vi "HGF_PVBase.appendData2Variant.vi"(0 "initData":variant, 2 "HGF_PVDataConverter":refnum<class "HGF_PVDataConverter.lvclass">, 5 "error in (no error)":errorcluster) -> (14 "dup initData":variant, 19 "error out":errorcluster)   [LabVIEW 2014, in "HGF_BaseClasses.lvlib" / "HGF_PVBase.lvclass"]
uses:
  HGF_PVBase.lvclass
  HGF_PVDataConverter/HGF_PVDataConverter.lvclass
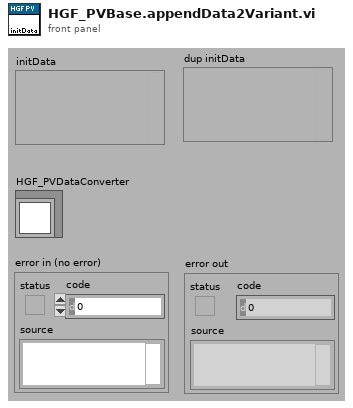
[diagram p1: front panel]
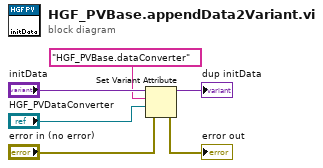
[diagram p0: block diagram]
diagram:
  n1 = Set Variant Attribute(Variant="initData", name="HGF_PVBase.dataConverter", value="HGF_PVDataConverter", error in="error in (no error)") -> (Variant out=→"dup initData":variant, error out=→"error out":errorcluster)  [unwired: 1 out]
